vi "Stop Core.vi"(10 "final error code":i32, 11 "CS++OPCUAInterface in":refnum<class "CS++OPCUAInterface.lvclass">) -> (3 "CS++OPCUAInterface out":refnum<class "CS++OPCUAInterface.lvclass">)   [LabVIEW 2016, in "CS++OPCUAInterface.lvlib" / "CS++OPCUAInterface.lvclass"]
doc: "(<B>Filename</B>: Actor Framework.lvlib:Actor.lvclass:Stop Core.vi)\n\nDefines what the actor does before it stops. Use the <B>final error code</B> input to determine whether the actor shut down in response to an error.\n\nBy default, this method does nothing. A descendant class may override it to define behavior, such as shutting down any processes the actor initiated in its override of the Actor Core method."
uses:
  CS++OPCUAInterface.lvclass
  CS++OPCUAInterface.lvclass/CS++OPCUAInterface.ctl
  <vilib>/event_ctls.llb/usereventprio.ctl
  <vilib>/ActorFramework/Stop Msg/Stop Msg.lvclass/Stop Msg.ctl
  <vilib>/ActorFramework/Message Enqueuer/Message Enqueuer.lvclass/Message Enqueuer.ctl
  <vilib>/ActorFramework/Message Enqueuer/Enqueue Critical.vi
  <vilib>/ActorFramework/Stop Msg/Stop Msg.lvclass
  C:/Program Files (x86)/National Instruments/LabVIEW 2016/vi.lib/ActorFramework/Message/Message.lvclass
  <vilib>/ActorFramework/Message Priority Queue/Priority Enqueue.vi
  CSPP_Core/Actors/CS++BaseActor/CS++BaseActor.lvclass
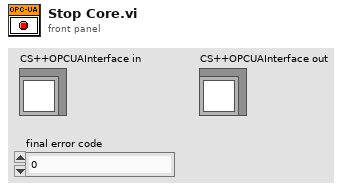
[diagram p1: front panel]
types:
  T1 = typedef "usereventprio.ctl" = enum32{"high priority", "normal priority"}
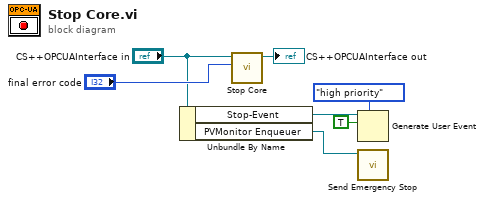
[diagram p0: block diagram]
diagram:
  n1 = Unbundle By Name("CS++OPCUAInterface in") -> ("Stop-Event"=w4:refnum<user-event>, "PVMonitor Enqueuer"=w1:refnum<class "Message Enqueuer.lvclass">)
  n2 = call-parent "Stop Core.vi"("final error code"="final error code", "CS++BaseActor in"="CS++OPCUAInterface in") -> ("CS++BaseActor out"=→"CS++OPCUAInterface out":refnum<class "CS++OPCUAInterface.lvclass">)  [unwired: 9 in]
  n3 = Generate User Event(priority (normal)=usereventprio."high priority", user event=w4, event data cluster=TRUE ("event data")) -> ()  [unwired: 1 in, 2 out]
  n4 = call <vilib>:"Send Emergency Stop.vi"("Message Enqueuer"=w1) -> ()  [unwired: 10 in, 1 out]
